vi "历史数据读取.vi"(4 "error in (no error)":errorcluster caption="错误输入（无错误）", 6 "Container State":T4 caption="容器状态", 7 "Display State In":T2={"完成"=FALSE, "功能选择"=enum."扫描", "数据"=[], "历史数据"=[], "曲线设置"={"X"=enum."设置电压", "Y1"=enum."读取电流", "Y2"=enum."无", "Y3"=enum."无"}, "突变电压"=refnum, "保留数量"=0, "属性"=variant} caption="显示状态输入") -> (0 "error out":errorcluster caption="错误输出", 2 "Value":T1[](array[typedef]) caption="历史数据", 3 "Display State Out":T2={"完成"=FALSE, "功能选择"=enum."扫描", "数据"=[], "历史数据"=[], "曲线设置"={"X"=enum."设置电压", "Y1"=enum."读取电流", "Y2"=enum."无", "Y3"=enum."无"}, "突变电压"=refnum, "保留数量"=0, "属性"=variant} caption="显示状态输出")   [LabVIEW 2020, in "数据显示.xctl"]
uses:
  <vilib>/_xctls/Container State.ctl
  <vilib>/_xctls/XControlSupport.lvlib
panel:
  # "将以下值显示控件替换为所需类型的显示控件。\n不要从连线板中删除该显示控件或其它显示控件。\n不要更改连线板模式。\n值显示控件应始终位于连线板输出端自顶部起第二个接线端。"
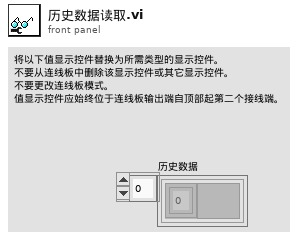
[diagram p1: front panel]
types:
  T1 = typedef "数据显示.xctl/波形数据定义.ctl" = cluster{"波形":dbl[][], "属性":variant}
  T2 = typedef "数据显示.xctl/状态.ctl" = cluster{"完成":bool, "功能选择":enum16{"扫描", "循环扫描", "保持时间", "脉冲", "高速脉冲", "任意波形"}, "数据":dbl[][], "历史数据":T1[], "曲线设置":T3, "突变电压":refnum<user-event>, "保留数量":i32, "属性":variant}
  T3 = typedef "数据显示.xctl/曲线设置.ctl" = cluster{"X":enum16{"时间", "设置电压", "读取电流", "读取电压"}, "Y1":enum16{"时间", "设置电压", "读取电流", "读取电压"}, "Y2":enum16{"时间", "设置电压", "读取电流", "读取电压", "无"}, "Y3":enum16{"时间", "设置电压", "读取电流", "读取电压", "无"}}
  T4 = typedef "XControlSupport.lvlib/Container State.ctl" = cluster{"Indicator?":bool, "Run Mode?":bool, " Refnum":refnum<vi>}
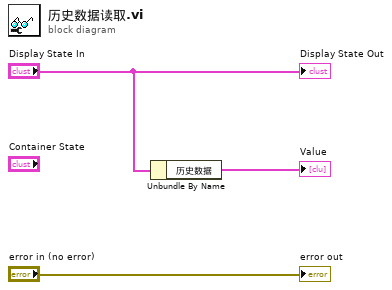
[diagram p0: block diagram]
diagram:
  n1 = Unbundle By Name("Display State In") -> ("历史数据"=→"Value":T1[])
  "error out" <- "error in (no error)"
  "Display State Out" <- "Display State In"
